vi "Main Rio.vi"() -> ()   [LabVIEW 2015]
uses:
  <vilib>/myRIO/Instrument Drivers/Onboard IO/DIO/typedefs/DIO Reference.ctl
  <vilib>/myRIO/Common/Instrument Driver Framework/Utilities/typedefs/myRIO Generic Hardware Reference.ctl
  <vilib>/myRIO/Common/Instrument Driver Framework/Utilities/typedefs/Hardware Version Enum.ctl
  <vilib>/myRIO/Common/Instrument Driver Framework/Utilities/typedefs/myRIO v1.0 Reference.ctl
  <vilib>/myRIO/Common/Instrument Driver Framework/Utilities/typedefs/Generic FPGA Reference.ctl
  <vilib>/myRIO/Common/Instrument Driver Framework/myRIO v1.0/DIO/typedefs/DIO Channels List.ctl
  <vilib>/myRIO/Common/Instrument Driver Framework/myRIO v1.0/DIO/typedefs/DIO Channels Enum.ctl
  <vilib>/userdefined/High Color/nirio_resource_hc.ctl
  <vilib>/myRIO/Instrument Drivers/Onboard IO/UART/typedef/VISA Configuration.ctl
  <vilib>/myRIO/Common/Instrument Driver Framework/Utilities/vis/Is FPGA Ref Available.vi
  <vilib>/myRIO/Common/Instrument Driver Framework/myRIO v1.0/DIO/vis/myRIO v1.1 Open DIO.vi
  <vilib>/myRIO/Instrument Drivers/Onboard IO/DIO/vis/Write.vi
  <vilib>/myRIO/Common/Instrument Driver Framework/Utilities/vis/Validate Channels.vi
  <vilib>/myRIO/Common/Instrument Driver Framework/myRIO v1.0/DIO/vis/myRIO v1.0 Reserve DIO.vi
  <vilib>/myRIO/Common/Instrument Driver Framework/myRIO v1.0/Resource Manager/vis/myRIO v1.0 Reserve Channel List.vi
  <vilib>/myRIO/Common/Instrument Driver Framework/myRIO v1.0/DIO/vis/myRIO v1.0 Build MUX Configuration DIO.vi
  <vilib>/myRIO/Common/Instrument Driver Framework/myRIO v1.0/Resource Manager/vis/myRIO v1.0 Reserve Channel.vi
  <vilib>/myRIO/Common/Instrument Driver Framework/myRIO v1.0/Resource Manager/vis/myRIO v1.0 Unreserve Channel.vi
  <vilib>/myRIO/Common/Instrument Driver Framework/myRIO v1.0/Resource Manager/vis/myRIO v1.0 Create Configuration List.vi
  <vilib>/myRIO/Common/Instrument Driver Framework/myRIO v1.0/Resource Manager/vis/myRIO v1.0 Build Mutex Name.vi
  <vilib>/Utility/VariantDataType/GetNumericInfo.vi
  <vilib>/Utility/error.llb/Error Cluster From Error Code.vi
  <vilib>/myRIO/Common/Instrument Driver Framework/myRIO v1.0/myRIO v1.1 Open.vi
  <vilib>/myRIO/Common/Instrument Driver Framework/Utilities/vis/IO Manager.vi
  <vilib>/myRIO/Common/Instrument Driver Framework/Utilities/vis/Configuration Manager.vi
  <vilib>/myRIO/Common/Instrument Driver Framework/myRIO v1.0/Resource Manager/vis/myRIO v1.0 Configure IO.vi
  <vilib>/myRIO/Common/Instrument Driver Framework/myRIO v1.0/myRIO v1.0 Close.vi
  <vilib>/myRIO/Common/Instrument Driver Framework/myRIO v1.0/DIO/vis/myRIO v1.0 Write DIO.vi
  <vilib>/Instr/_visa.llb/VISA Configure Serial Port (Instr).vi
  <vilib>/myRIO/Express VI/Onboard Devices/LED/LED Express VI.xnode
  <vilib>/myRIO/Instrument Drivers/Onboard IO/DIO/vis/myRIO DIO Open.xnode
  <vilib>/myRIO/Express VI/Onboard IO/UART/UART Express VI.xnode
  <vilib>/myRIO/Instrument Drivers/Onboard IO/UART/UART.lvlib
  <vilib>/myRIO/Instrument Drivers/Onboard IO/DIO/DIO.lvlib
panel:
  in  "Stop Button":bool
  out "KeyPress":dbl
  out "Consigne Mode":dbl
  # "Overview: The myRIO Project template acquires acceleration data from the onboard accelerometer and displays the changes of acceleration values in a waveform chart.\nInstructions:\n1. Check the myRIO target IP Address in the project and make sure the target IP Address is correct. \n2. Run the VI."
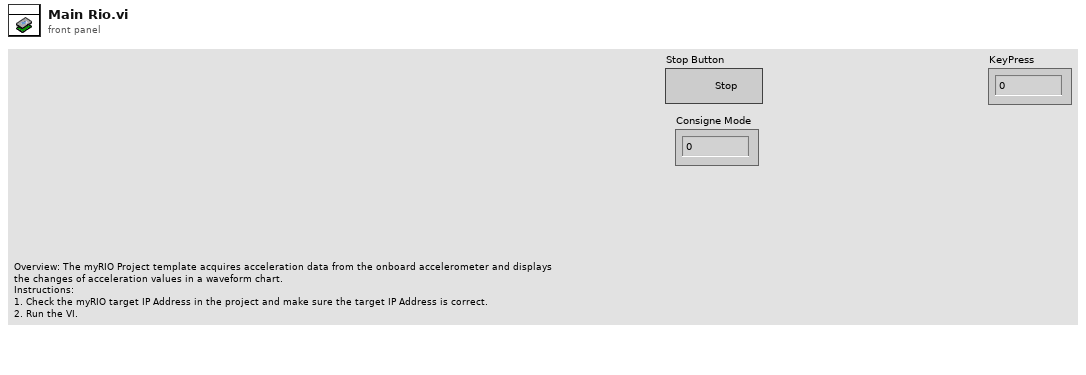
[diagram p1: front panel]
types:
  T1 = typedef "UART.lvlib/VISA Configuration.ctl" = cluster{"baud rate (9600)":u32, "data bits (8)":u16, "parity (0:none)":enum16{"None", "Odd", "Even", "Mark", "Space"}, "stop bits (10: 1 bit)":u16, "flow control (0:none)":u16, "termination char\n(0xA = '\\n' = LF) ":u8, "Enable Termination\nChar (T)":bool, "timeout (10sec)":u32}
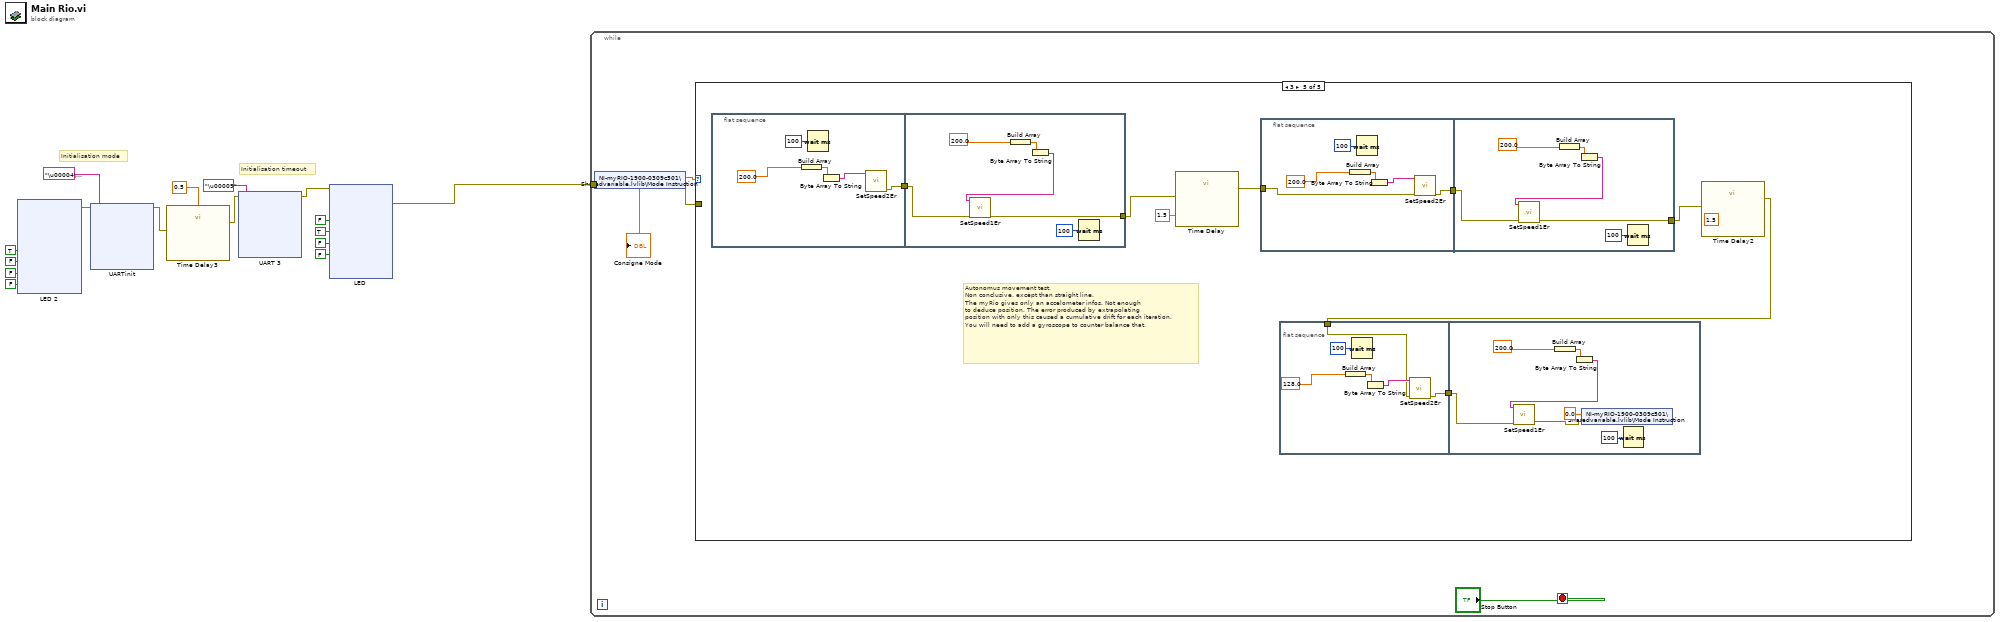
[diagram p0: block diagram]
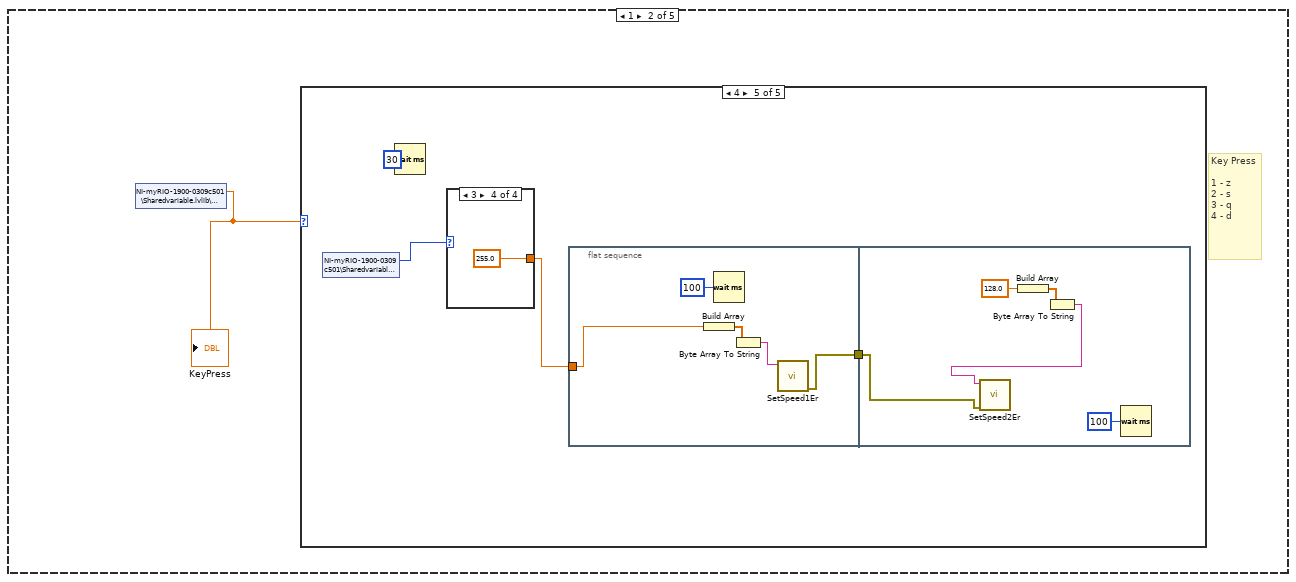
[diagram p3: hidden frame]
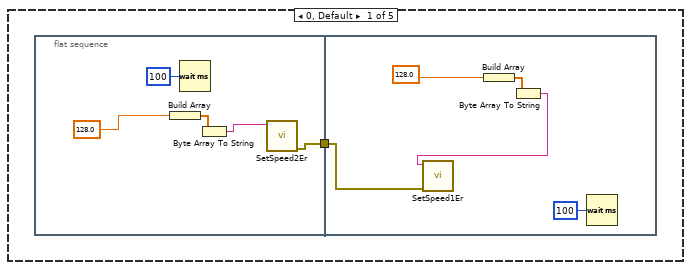
[diagram p4: hidden frame]
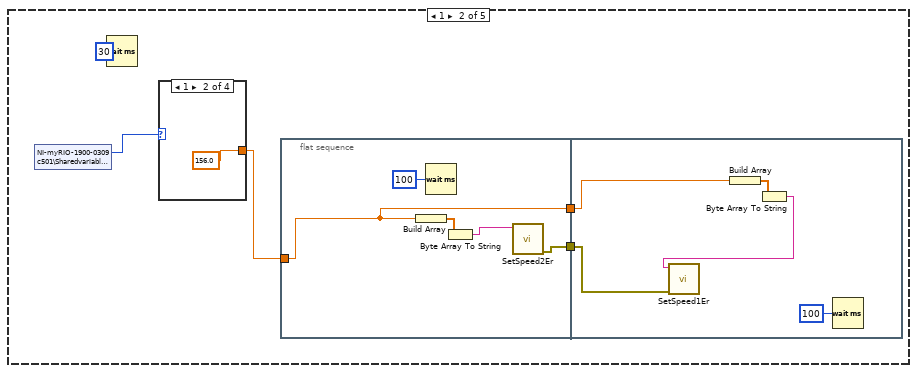
[diagram p5: hidden frame]
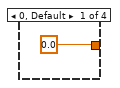
[diagram p6: hidden frame]
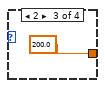
[diagram p7: hidden frame]
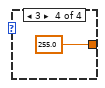
[diagram p8: hidden frame]
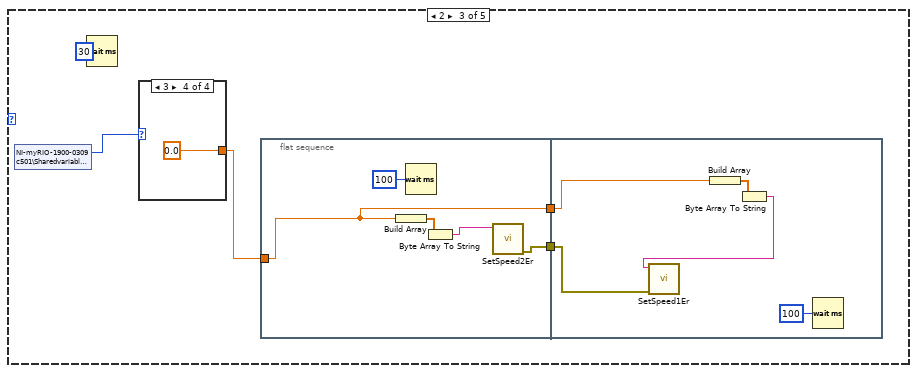
[diagram p9: hidden frame]
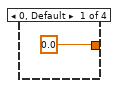
[diagram p10: hidden frame]
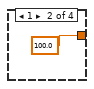
[diagram p11: hidden frame]
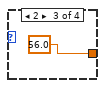
[diagram p12: hidden frame]
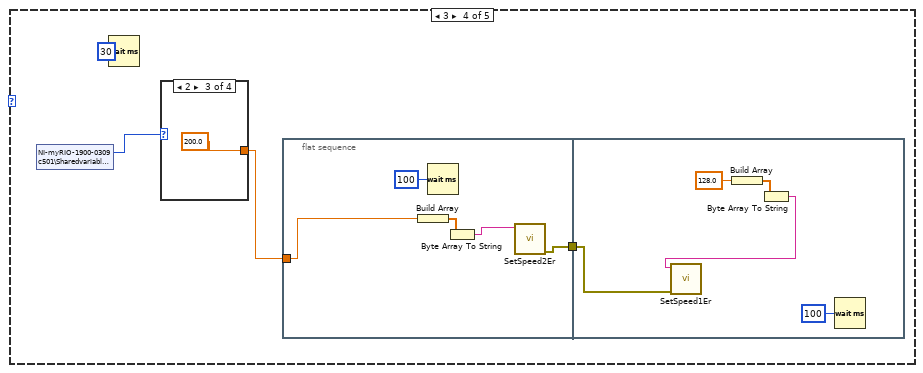
[diagram p13: hidden frame]
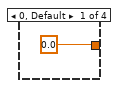
[diagram p14: hidden frame]
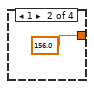
[diagram p15: hidden frame]
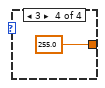
[diagram p16: hidden frame]
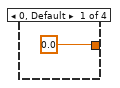
[diagram p17: hidden frame]
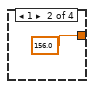
[diagram p18: hidden frame]
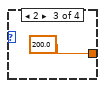
[diagram p19: hidden frame]
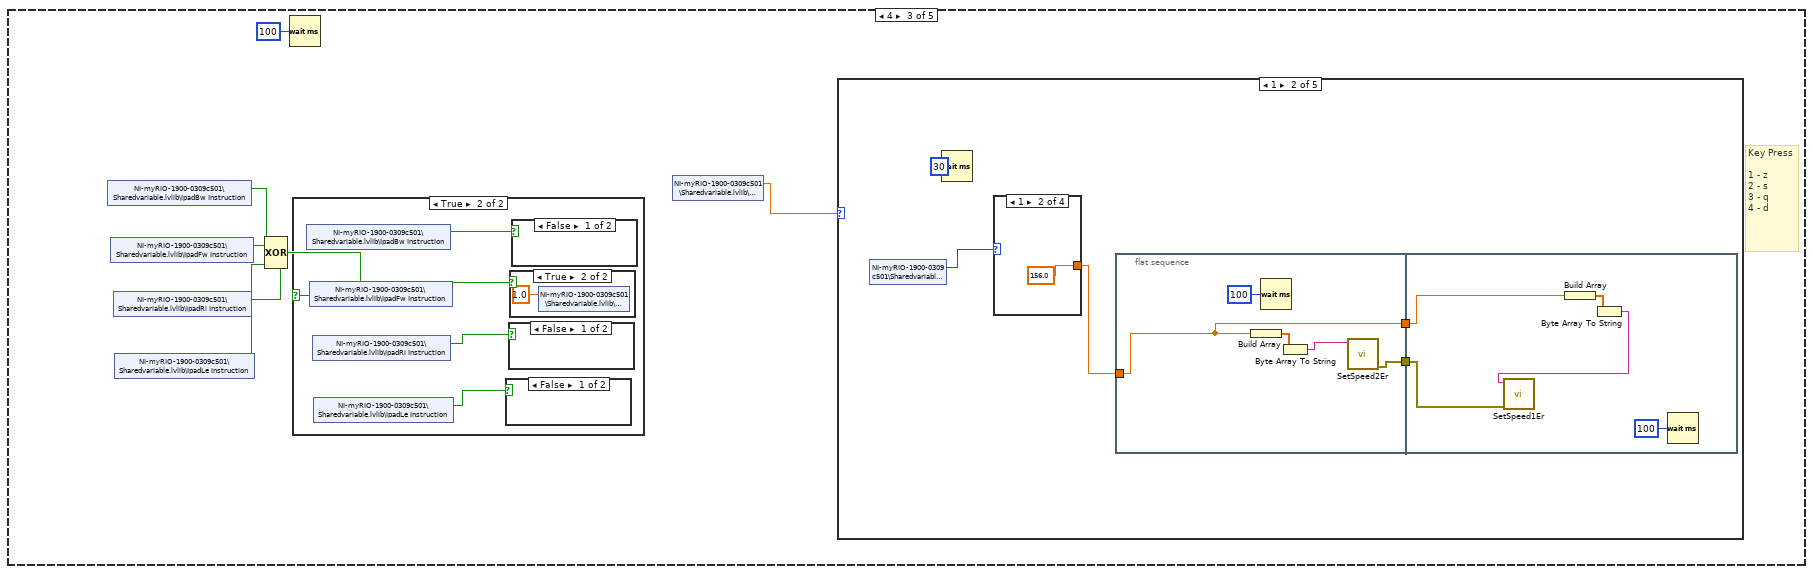
[diagram p20: hidden frame]
diagram:
  # "Initialisation timeout"
  # "Initialisation mode"
  n1 = xnode "LED 2"("LED0"=TRUE, "LED1"=FALSE, "LED2"=FALSE, "LED3"=FALSE) -> ("error out"=w10:errorcluster)  [unwired: 1 in]
  n2 = xnode "UARTinit"("Characters to Write"="\u00004\u0000", "error in (no error)"=w10) -> ("error out"=w2:errorcluster)  [unwired: 1 out]
  n3 = call "Time Delay3"("error in (no error)"=w2, "Delay Time (s)"=0.5) -> ("error out"=w1:errorcluster)  [unwired: 9 in]
  n4 = xnode "UART 3"("Characters to Write"="\u00009", "error in (no error)"=w1) -> ("error out"=w5:errorcluster)  [unwired: 1 out]
  n5 = xnode "LED"("LED0"=FALSE, "LED1"=TRUE, "LED2"=FALSE, "LED3"=FALSE, "error in (no error)"=w5) -> ("error out"=w4:errorcluster)
  n6 = while {
    tunnel: w4 -> [w17]
    stop <- "Stop Button" stop-if-true
    n7 = shared-variable "NI-myRIO-1900-0309c501\\Sharedvariable.lvlib\\Mode Instruction"(error in=w17) -> (w20:dbl, error out=w19:errorcluster)
    "Consigne Mode" <- w20
    n8 = case shown="3" w20 {
      tunnel: w19 -> [_ _ _ _ _]
      frame 0, Default {
      }
      frame 1 {
        # "Key Press\n\n1 - z\n2 - s\n3 - q\n4 - d"
        n9 = shared-variable "NI-myRIO-1900-0309c501\\Sharedvariable.lvlib\\KeyPress"() -> (w21:dbl)  [unwired: 1 in, 1 out]
        "KeyPress" <- w21
        n10 = case shown="4" w21 {
          frame 0, Default {
            n11 = flat-sequence {
              tunnel: [w25] -> w22
              tunnel: w22 -> [w30]
              frame #0 {
                n12 = Build Array(128.0 ("element")) -> (w27:dbl[])
                n13 = Wait (ms)(milliseconds to wait=u32 100) -> ()  [unwired: 1 out]
                n14 = Byte Array To String(unsigned byte array=w27) -> (string=w26:string)
                n15 = call "SetSpeed2Er.vi"("Chaîne en entrée"=w26) -> ("error out"=w25:errorcluster)  [unwired: 10 in]
              }
              frame #1 {
                n16 = Build Array(128.0 ("element")) -> (w32:dbl[])
                n17 = Byte Array To String(unsigned byte array=w32) -> (string=w31:string)
                n18 = call "SetSpeed1Er.vi"("error in (no error)"=w30, "Chaîne"=w31) -> ()  [unwired: 9 in, 1 out]
                n19 = Wait (ms)(milliseconds to wait=u32 100) -> ()  [unwired: 1 out]
              }
            }
          }
          frame 1 {
            n20 = shared-variable "NI-myRIO-1900-0309c501\\Sharedvariable.lvlib\\Speed"() -> (w37:u16)  [unwired: 1 in, 1 out]
            n21 = Wait (ms)(milliseconds to wait=u32 30) -> ()  [unwired: 1 out]
            n22 = case shown="1" w37 {
              tunnel: [0.0 156.0 200.0 255.0] -> w34
              frame 0, Default {
              }
              frame 1 {
              }
              frame 2 {
              }
              frame 3 {
              }
            }
            n23 = flat-sequence {
              tunnel: [w40] -> w35
              tunnel: w34 -> [w38]
              tunnel: [w38] -> w33
              tunnel: w35 -> [w45]
              tunnel: w33 -> [w43]
              frame #0 {
                n24 = Build Array(w38) -> (w42:dbl[])
                n25 = Wait (ms)(milliseconds to wait=u32 100) -> ()  [unwired: 1 out]
                n26 = Byte Array To String(unsigned byte array=w42) -> (string=w41:string)
                n27 = call "SetSpeed2Er.vi"("Chaîne en entrée"=w41) -> ("error out"=w40:errorcluster)  [unwired: 10 in]
              }
              frame #1 {
                n28 = Build Array(w43) -> (w47:dbl[])
                n29 = Byte Array To String(unsigned byte array=w47) -> (string=w46:string)
                n30 = call "SetSpeed1Er.vi"("error in (no error)"=w45, "Chaîne"=w46) -> ()  [unwired: 9 in, 1 out]
                n31 = Wait (ms)(milliseconds to wait=u32 100) -> ()  [unwired: 1 out]
              }
            }
          }
          frame 2 {
            n32 = shared-variable "NI-myRIO-1900-0309c501\\Sharedvariable.lvlib\\Speed"() -> (w54:u16)  [unwired: 1 in, 1 out]
            n33 = Wait (ms)(milliseconds to wait=u32 30) -> ()  [unwired: 1 out]
            n34 = case shown="3" w54 {
              tunnel: [0.0 100.0 56.0 0.0] -> w52
              frame 0, Default {
              }
              frame 1 {
              }
              frame 2 {
              }
              frame 3 {
              }
            }
            n35 = flat-sequence {
              tunnel: [w59] -> w56
              tunnel: w52 -> [w57]
              tunnel: [w57] -> w55
              tunnel: w56 -> [w64]
              tunnel: w55 -> [w62]
              frame #0 {
                n36 = Build Array(w57) -> (w61:dbl[])
                n37 = Wait (ms)(milliseconds to wait=u32 100) -> ()  [unwired: 1 out]
                n38 = Byte Array To String(unsigned byte array=w61) -> (string=w60:string)
                n39 = call "SetSpeed2Er.vi"("Chaîne en entrée"=w60) -> ("error out"=w59:errorcluster)  [unwired: 10 in]
              }
              frame #1 {
                n40 = Build Array(w62) -> (w66:dbl[])
                n41 = Byte Array To String(unsigned byte array=w66) -> (string=w65:string)
                n42 = call "SetSpeed1Er.vi"("error in (no error)"=w64, "Chaîne"=w65) -> ()  [unwired: 9 in, 1 out]
                n43 = Wait (ms)(milliseconds to wait=u32 100) -> ()  [unwired: 1 out]
              }
            }
          }
          frame 3 {
            n44 = shared-variable "NI-myRIO-1900-0309c501\\Sharedvariable.lvlib\\Speed"() -> (w73:u16)  [unwired: 1 in, 1 out]
            n45 = Wait (ms)(milliseconds to wait=u32 30) -> ()  [unwired: 1 out]
            n46 = case shown="2" w73 {
              tunnel: [0.0 156.0 200.0 255.0] -> w71
              frame 0, Default {
              }
              frame 1 {
              }
              frame 2 {
              }
              frame 3 {
              }
            }
            n47 = flat-sequence {
              tunnel: [w77] -> w74
              tunnel: w71 -> [w75]
              tunnel: w74 -> [w82]
              frame #0 {
                n48 = Build Array(w75) -> (w79:dbl[])
                n49 = Wait (ms)(milliseconds to wait=u32 100) -> ()  [unwired: 1 out]
                n50 = Byte Array To String(unsigned byte array=w79) -> (string=w78:string)
                n51 = call "SetSpeed2Er.vi"("Chaîne en entrée"=w78) -> ("error out"=w77:errorcluster)  [unwired: 10 in]
              }
              frame #1 {
                n52 = Build Array(128.0 ("element")) -> (w84:dbl[])
                n53 = Byte Array To String(unsigned byte array=w84) -> (string=w83:string)
                n54 = call "SetSpeed1Er.vi"("error in (no error)"=w82, "Chaîne"=w83) -> ()  [unwired: 9 in, 1 out]
                n55 = Wait (ms)(milliseconds to wait=u32 100) -> ()  [unwired: 1 out]
              }
            }
          }
          frame 4 {
            n56 = shared-variable "NI-myRIO-1900-0309c501\\Sharedvariable.lvlib\\Speed"() -> (w91:u16)  [unwired: 1 in, 1 out]
            n57 = Wait (ms)(milliseconds to wait=u32 30) -> ()  [unwired: 1 out]
            n58 = case shown="3" w91 {
              tunnel: [0.0 156.0 200.0 255.0] -> w89
              frame 0, Default {
              }
              frame 1 {
              }
              frame 2 {
              }
              frame 3 {
              }
            }
            n59 = flat-sequence {
              tunnel: [w93] -> w92
              tunnel: w89 -> [w95]
              tunnel: w92 -> [w98]
              frame #0 {
                n60 = Build Array(w95) -> (w97:dbl[])
                n61 = Wait (ms)(milliseconds to wait=u32 100) -> ()  [unwired: 1 out]
                n62 = Byte Array To String(unsigned byte array=w97) -> (string=w94:string)
                n63 = call "SetSpeed1Er.vi"("Chaîne"=w94) -> ("error out"=w93:errorcluster)  [unwired: 10 in]
              }
              frame #1 {
                n64 = Build Array(128.0 ("element")) -> (w102:dbl[])
                n65 = Byte Array To String(unsigned byte array=w102) -> (string=w99:string)
                n66 = call "SetSpeed2Er.vi"("error in (no error)"=w98, "Chaîne en entrée"=w99) -> ()  [unwired: 9 in, 1 out]
                n67 = Wait (ms)(milliseconds to wait=u32 100) -> ()  [unwired: 1 out]
              }
            }
          }
        }
      }
      frame 4 {
        # "Key Press\n\n1 - z\n2 - s\n3 - q\n4 - d"
        n68 = shared-variable "NI-myRIO-1900-0309c501\\Sharedvariable.lvlib\\IpadBw Instruction"() -> (w113:bool)  [unwired: 1 in, 1 out]
        n69 = shared-variable "NI-myRIO-1900-0309c501\\Sharedvariable.lvlib\\IpadFw Instruction"() -> (w112:bool)  [unwired: 1 in, 1 out]
        n70 = shared-variable "NI-myRIO-1900-0309c501\\Sharedvariable.lvlib\\IpadRi Instruction"() -> (w111:bool)  [unwired: 1 in, 1 out]
        n71 = shared-variable "NI-myRIO-1900-0309c501\\Sharedvariable.lvlib\\IpadLe Instruction"() -> (w110:bool)  [unwired: 1 in, 1 out]
        n72 = Compound Arithmetic op=XOR(w113, w112, w111, w110) -> (w109:bool)
        n73 = Wait (ms)(milliseconds to wait=u32 100) -> ()  [unwired: 1 out]
        n74 = case shown="True" w109 {
          frame False {
            n75 = shared-variable "NI-myRIO-1900-0309c501\\Sharedvariable.lvlib\\IpadBw Instruction"(FALSE ("Consigne ArIpad")) -> ()  [unwired: 1 in, 1 out]
            n76 = shared-variable "NI-myRIO-1900-0309c501\\Sharedvariable.lvlib\\IpadFw Instruction"(FALSE ("Consigne AvIpad")) -> ()  [unwired: 1 in, 1 out]
            n77 = shared-variable "NI-myRIO-1900-0309c501\\Sharedvariable.lvlib\\IpadRi Instruction"(FALSE ("Consigne DroiIpad")) -> ()  [unwired: 1 in, 1 out]
            n78 = shared-variable "NI-myRIO-1900-0309c501\\Sharedvariable.lvlib\\IpadLe Instruction"(FALSE ("Consigne GauIpad")) -> ()  [unwired: 1 in, 1 out]
            n79 = shared-variable "NI-myRIO-1900-0309c501\\Sharedvariable.lvlib\\KeyPress"(0.0 ("KeyPress")) -> ()  [unwired: 1 in, 1 out]
          }
          frame True {
            n80 = shared-variable "NI-myRIO-1900-0309c501\\Sharedvariable.lvlib\\IpadBw Instruction"() -> (w207:bool)  [unwired: 1 in, 1 out]
            n81 = shared-variable "NI-myRIO-1900-0309c501\\Sharedvariable.lvlib\\IpadFw Instruction"() -> (w206:bool)  [unwired: 1 in, 1 out]
            n82 = shared-variable "NI-myRIO-1900-0309c501\\Sharedvariable.lvlib\\IpadRi Instruction"() -> (w205:bool)  [unwired: 1 in, 1 out]
            n83 = shared-variable "NI-myRIO-1900-0309c501\\Sharedvariable.lvlib\\IpadLe Instruction"() -> (w204:bool)  [unwired: 1 in, 1 out]
            n84 = case shown="False" w204 {
              frame False {
              }
              frame True {
                n85 = shared-variable "NI-myRIO-1900-0309c501\\Sharedvariable.lvlib\\KeyPress"(3.0 ("KeyPress")) -> ()  [unwired: 1 in, 1 out]
              }
            }
            n86 = case shown="False" w205 {
              frame False {
              }
              frame True {
                n87 = shared-variable "NI-myRIO-1900-0309c501\\Sharedvariable.lvlib\\KeyPress"(4.0 ("KeyPress")) -> ()  [unwired: 1 in, 1 out]
              }
            }
            n88 = case shown="True" w206 {
              frame False {
              }
              frame True {
                n89 = shared-variable "NI-myRIO-1900-0309c501\\Sharedvariable.lvlib\\KeyPress"(1.0 ("KeyPress")) -> ()  [unwired: 1 in, 1 out]
              }
            }
            n90 = case shown="False" w207 {
              frame False {
              }
              frame True {
                n91 = shared-variable "NI-myRIO-1900-0309c501\\Sharedvariable.lvlib\\KeyPress"(2.0 ("KeyPress")) -> ()  [unwired: 1 in, 1 out]
              }
            }
          }
        }
        n92 = shared-variable "NI-myRIO-1900-0309c501\\Sharedvariable.lvlib\\KeyPress"() -> (w107:dbl)  [unwired: 1 in, 1 out]
        n93 = case shown="1" w107 {
          frame 0, Default {
            n94 = flat-sequence {
              tunnel: [w117] -> w114
              tunnel: w114 -> [w122]
              frame #0 {
                n95 = Build Array(128.0 ("element")) -> (w119:dbl[])
                n96 = Wait (ms)(milliseconds to wait=u32 100) -> ()  [unwired: 1 out]
                n97 = Byte Array To String(unsigned byte array=w119) -> (string=w118:string)
                n98 = call "SetSpeed2Er.vi"("Chaîne en entrée"=w118) -> ("error out"=w117:errorcluster)  [unwired: 10 in]
              }
              frame #1 {
                n99 = Build Array(128.0 ("element")) -> (w124:dbl[])
                n100 = Byte Array To String(unsigned byte array=w124) -> (string=w123:string)
                n101 = call "SetSpeed1Er.vi"("error in (no error)"=w122, "Chaîne"=w123) -> ()  [unwired: 9 in, 1 out]
                n102 = Wait (ms)(milliseconds to wait=u32 100) -> ()  [unwired: 1 out]
              }
            }
          }
          frame 1 {
            n103 = shared-variable "NI-myRIO-1900-0309c501\\Sharedvariable.lvlib\\Speed"() -> (w129:u16)  [unwired: 1 in, 1 out]
            n104 = Wait (ms)(milliseconds to wait=u32 30) -> ()  [unwired: 1 out]
            n105 = case shown="1" w129 {
              tunnel: [0.0 156.0 200.0 255.0] -> w126
              frame 0, Default {
              }
              frame 1 {
              }
              frame 2 {
              }
              frame 3 {
              }
            }
            n106 = flat-sequence {
              tunnel: [w132] -> w127
              tunnel: w126 -> [w130]
              tunnel: [w130] -> w125
              tunnel: w127 -> [w137]
              tunnel: w125 -> [w135]
              frame #0 {
                n107 = Build Array(w130) -> (w134:dbl[])
                n108 = Wait (ms)(milliseconds to wait=u32 100) -> ()  [unwired: 1 out]
                n109 = Byte Array To String(unsigned byte array=w134) -> (string=w133:string)
                n110 = call "SetSpeed2Er.vi"("Chaîne en entrée"=w133) -> ("error out"=w132:errorcluster)  [unwired: 10 in]
              }
              frame #1 {
                n111 = Build Array(w135) -> (w139:dbl[])
                n112 = Byte Array To String(unsigned byte array=w139) -> (string=w138:string)
                n113 = call "SetSpeed1Er.vi"("error in (no error)"=w137, "Chaîne"=w138) -> ()  [unwired: 9 in, 1 out]
                n114 = Wait (ms)(milliseconds to wait=u32 100) -> ()  [unwired: 1 out]
              }
            }
          }
          frame 2 {
            n115 = shared-variable "NI-myRIO-1900-0309c501\\Sharedvariable.lvlib\\Speed"() -> (w146:u16)  [unwired: 1 in, 1 out]
            n116 = Wait (ms)(milliseconds to wait=u32 30) -> ()  [unwired: 1 out]
            n117 = case shown="3" w146 {
              tunnel: [0.0 100.0 56.0 0.0] -> w144
              frame 0, Default {
              }
              frame 1 {
              }
              frame 2 {
              }
              frame 3 {
              }
            }
            n118 = flat-sequence {
              tunnel: [w151] -> w148
              tunnel: w144 -> [w149]
              tunnel: [w149] -> w147
              tunnel: w148 -> [w156]
              tunnel: w147 -> [w154]
              frame #0 {
                n119 = Build Array(w149) -> (w153:dbl[])
                n120 = Wait (ms)(milliseconds to wait=u32 100) -> ()  [unwired: 1 out]
                n121 = Byte Array To String(unsigned byte array=w153) -> (string=w152:string)
                n122 = call "SetSpeed2Er.vi"("Chaîne en entrée"=w152) -> ("error out"=w151:errorcluster)  [unwired: 10 in]
              }
              frame #1 {
                n123 = Build Array(w154) -> (w158:dbl[])
                n124 = Byte Array To String(unsigned byte array=w158) -> (string=w157:string)
                n125 = call "SetSpeed1Er.vi"("error in (no error)"=w156, "Chaîne"=w157) -> ()  [unwired: 9 in, 1 out]
                n126 = Wait (ms)(milliseconds to wait=u32 100) -> ()  [unwired: 1 out]
              }
            }
          }
          frame 3 {
            n127 = shared-variable "NI-myRIO-1900-0309c501\\Sharedvariable.lvlib\\Speed"() -> (w165:u16)  [unwired: 1 in, 1 out]
            n128 = Wait (ms)(milliseconds to wait=u32 30) -> ()  [unwired: 1 out]
            n129 = case shown="3" w165 {
              tunnel: [0.0 156.0 200.0 255.0] -> w163
              frame 0, Default {
              }
              frame 1 {
              }
              frame 2 {
              }
              frame 3 {
              }
            }
            n130 = flat-sequence {
              tunnel: [w169] -> w166
              tunnel: w163 -> [w167]
              tunnel: w166 -> [w174]
              frame #0 {
                n131 = Build Array(w167) -> (w171:dbl[])
                n132 = Wait (ms)(milliseconds to wait=u32 100) -> ()  [unwired: 1 out]
                n133 = Byte Array To String(unsigned byte array=w171) -> (string=w170:string)
                n134 = call "SetSpeed2Er.vi"("Chaîne en entrée"=w170) -> ("error out"=w169:errorcluster)  [unwired: 10 in]
              }
              frame #1 {
                n135 = Build Array(128.0 ("element")) -> (w176:dbl[])
                n136 = Byte Array To String(unsigned byte array=w176) -> (string=w175:string)
                n137 = call "SetSpeed1Er.vi"("error in (no error)"=w174, "Chaîne"=w175) -> ()  [unwired: 9 in, 1 out]
                n138 = Wait (ms)(milliseconds to wait=u32 100) -> ()  [unwired: 1 out]
              }
            }
          }
          frame 4 {
            n139 = shared-variable "NI-myRIO-1900-0309c501\\Sharedvariable.lvlib\\Speed"() -> (w183:u16)  [unwired: 1 in, 1 out]
            n140 = Wait (ms)(milliseconds to wait=u32 30) -> ()  [unwired: 1 out]
            n141 = case shown="3" w183 {
              tunnel: [0.0 156.0 200.0 255.0] -> w181
              frame 0, Default {
              }
              frame 1 {
              }
              frame 2 {
              }
              frame 3 {
              }
            }
            n142 = flat-sequence {
              tunnel: [w185] -> w184
              tunnel: w181 -> [w187]
              tunnel: w184 -> [w190]
              frame #0 {
                n143 = Build Array(w187) -> (w189:dbl[])
                n144 = Wait (ms)(milliseconds to wait=u32 100) -> ()  [unwired: 1 out]
                n145 = Byte Array To String(unsigned byte array=w189) -> (string=w186:string)
                n146 = call "SetSpeed1Er.vi"("Chaîne"=w186) -> ("error out"=w185:errorcluster)  [unwired: 10 in]
              }
              frame #1 {
                n147 = Build Array(128.0 ("element")) -> (w194:dbl[])
                n148 = Byte Array To String(unsigned byte array=w194) -> (string=w191:string)
                n149 = call "SetSpeed2Er.vi"("error in (no error)"=w190, "Chaîne en entrée"=w191) -> ()  [unwired: 9 in, 1 out]
                n150 = Wait (ms)(milliseconds to wait=u32 100) -> ()  [unwired: 1 out]
              }
            }
          }
        }
      }
      frame 2 {
        n151 = shared-variable "NI-myRIO-1900-0309c501\\Sharedvariable.lvlib\\Trame envoie"() -> (w217:string)  [unwired: 1 in, 1 out]
        n152 = xnode "UART"("Characters to Write"=w217) -> ("error out"=w212:errorcluster)  [unwired: 1 in, 1 out]
        n153 = xnode "UART 2"("error in (no error)"=w212) -> ("Characters Read"=w213:string)  [unwired: 1 out]
        n154 = Wait (ms)(milliseconds to wait=u32 50) -> ()  [unwired: 1 out]
        n155 = Not Equal?(x="", y=w213) -> (x != y?=w215:bool)
        n156 = case shown="True" w215 {
          tunnel: w213 -> [_ w218]
          frame False {
          }
          frame True {
            n157 = shared-variable "NI-myRIO-1900-0309c501\\Sharedvariable.lvlib\\Trame Recue"(w218) -> ()  [unwired: 1 in, 1 out]
          }
        }
      }
      frame 3 {
        # "Autonomus movement test,\nNon conclusive, except than straight line.\nThe myRio gives only an accelometer infos. Not enough \nto deduce position. The error produced by extrapolating\nposition with only this caused a cumulative drift for each iteration.\nYou will need to add a gyroscope to counter balance that."
        n158 = flat-sequence {
          tunnel: [w288] -> w260
          tunnel: w260 -> [w294]
          tunnel: [w291] -> w257
          frame #0 {
            n159 = Build Array(200.0 ("element")) -> (w290:dbl[])
            n160 = Wait (ms)(milliseconds to wait=u32 100) -> ()  [unwired: 1 out]
            n161 = Byte Array To String(unsigned byte array=w290) -> (string=w289:string)
            n162 = call "SetSpeed2Er.vi"("Chaîne en entrée"=w289) -> ("error out"=w288:errorcluster)  [unwired: 10 in]
          }
          frame #1 {
            n163 = Build Array(200.0 ("element")) -> (w296:dbl[])
            n164 = Byte Array To String(unsigned byte array=w296) -> (string=w295:string)
            n165 = call "SetSpeed1Er.vi"("error in (no error)"=w294, "Chaîne"=w295) -> ("error out"=w291:errorcluster)  [unwired: 9 in]
            n166 = Wait (ms)(milliseconds to wait=u32 100) -> ()  [unwired: 1 out]
          }
        }
        n167 = call "Time Delay"("error in (no error)"=w257, "Delay Time (s)"=1.5) -> ("error out"=w255:errorcluster)  [unwired: 9 in]
        n168 = flat-sequence {
          tunnel: [w264] -> w258
          tunnel: w255 -> [w261]
          tunnel: w258 -> [w270]
          tunnel: [w267] -> w256
          frame #0 {
            n169 = Build Array(200.0 ("element")) -> (w266:dbl[])
            n170 = Wait (ms)(milliseconds to wait=u32 100) -> ()  [unwired: 1 out]
            n171 = Byte Array To String(unsigned byte array=w266) -> (string=w265:string)
            n172 = call "SetSpeed2Er.vi"("error in (no error)"=w261, "Chaîne en entrée"=w265) -> ("error out"=w264:errorcluster)  [unwired: 9 in]
          }
          frame #1 {
            n173 = Build Array(200.0 ("element")) -> (w272:dbl[])
            n174 = Byte Array To String(unsigned byte array=w272) -> (string=w271:string)
            n175 = call "SetSpeed1Er.vi"("error in (no error)"=w270, "Chaîne"=w271) -> ("error out"=w267:errorcluster)  [unwired: 9 in]
            n176 = Wait (ms)(milliseconds to wait=u32 100) -> ()  [unwired: 1 out]
          }
        }
        n177 = flat-sequence {
          tunnel: [w276] -> w259
          tunnel: w252 -> [w273]
          tunnel: w259 -> [w283]
          frame #0 {
            n178 = Build Array(128.0 ("element")) -> (w278:dbl[])
            n179 = Wait (ms)(milliseconds to wait=u32 100) -> ()  [unwired: 1 out]
            n180 = Byte Array To String(unsigned byte array=w278) -> (string=w277:string)
            n181 = call "SetSpeed2Er.vi"("error in (no error)"=w273, "Chaîne en entrée"=w277) -> ("error out"=w276:errorcluster)  [unwired: 9 in]
          }
          frame #1 {
            n182 = Build Array(200.0 ("element")) -> (w285:dbl[])
            n183 = Byte Array To String(unsigned byte array=w285) -> (string=w284:string)
            n184 = call "SetSpeed1Er.vi"("error in (no error)"=w283, "Chaîne"=w284) -> ("error out"=w279:errorcluster)  [unwired: 9 in]
            n185 = shared-variable "NI-myRIO-1900-0309c501\\Sharedvariable.lvlib\\Mode Instruction"(0.0 ("Consigne Mode"), error in=w279) -> ()  [unwired: 1 out]
            n186 = Wait (ms)(milliseconds to wait=u32 100) -> ()  [unwired: 1 out]
          }
        }
        n187 = call "Time Delay2"("error in (no error)"=w256, "Delay Time (s)"=1.5) -> ("error out"=w252:errorcluster)  [unwired: 9 in]
      }
    }
  }
